vi "ADC_calc_samples_per_channel.vi"(2 "Samplingrate":dbl, 3 "Nchannel":dbl, 4 "time per point (ms)":dbl) -> (0 "effective samplingrate":dbl, 1 "samples to read":u32)   [LabVIEW 2013]
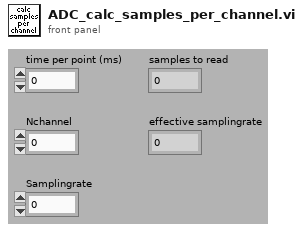
[diagram p1: front panel]
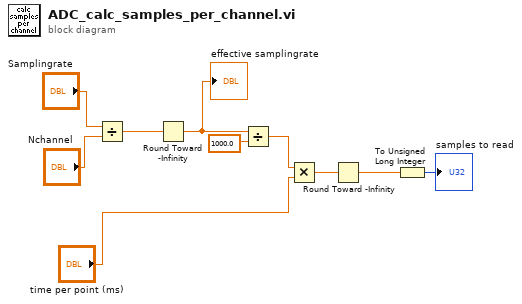
[diagram p0: block diagram]
diagram:
  n1 = Divide(x="Samplingrate", y="Nchannel") -> (x/y=w3:dbl)
  n2 = Round Toward -Infinity(1:w3) -> (0:w8:dbl)
  "effective samplingrate" <- w8
  n3 = Divide(x=w8, y=1000.0) -> (x/y=w9:dbl)
  n4 = Multiply(x=w9, y="time per point (ms)") -> (x*y=w6:dbl)
  n5 = Round Toward -Infinity(1:w6) -> (0:w1:dbl)
  n6 = To Unsigned Long Integer(number=w1) -> (unsigned 32bit integer=→"samples to read":u32)
